vi "Check Settings.vi"(8 "error in (no error)":errorcluster, 10 "Iterator Settings":T1={"Prepare timeout (ms)"=200, "Iterate timeout (ms)"=50, "Conclude timeout (ms)"=200, "Iterate period (ms)"=200, "Number of iterations"=5, "Stop Condition"=enum."None", "Time before stop (ms)"=5, "Prepare Msg"=refnum, "Iterate Msg"=refnum, "Conclude Msg"=refnum, "Error Handler"=refnum}, 11 "Caller Enqueuer in":refnum<class "Message Enqueuer.lvclass">) -> (0 "error out":errorcluster, 3 "Caller Enqueuer out":refnum<class "Message Enqueuer.lvclass">)   [LabVIEW 2016, in "Iterator Actor.lvlib" / "Iterator Actor.lvclass"]
doc: "Checks the input settings of the iterator. \nReturns an error with a description if something is wrong."
uses:
  Iterator Actor.lvclass
  <vilib>/ActorFramework/Message Enqueuer/Message Enqueuer.lvclass
  Iterator Settings.ctl
  Iterator Actor Abstract Messages/Iterator Reply Msg/Iterator Reply Msg.lvclass
  Iterator Actor Abstract Messages/Iterator Report Error Msg/Iterator Report Error Msg.lvclass
  Stop Condition.ctl
  Iterator Errors.ctl
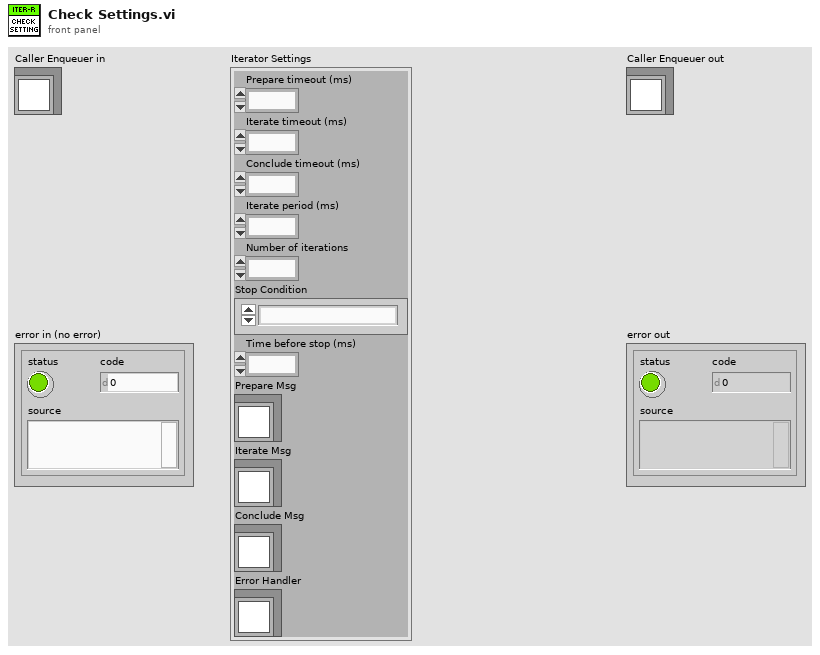
[diagram p1: front panel]
types:
  T1 = typedef "Iterator Actor.lvlib/Iterator Actor.lvclass/Iterator Settings.ctl" = cluster{"Prepare timeout (ms)":i32, "Iterate timeout (ms)":i32, "Conclude timeout (ms)":i32, "Iterate period (ms)":i32, "Number of iterations":i32, "Stop Condition":T2, "Time before stop (ms)":i32, "Prepare Msg":refnum<class "Iterator Reply Msg.lvclass">, "Iterate Msg":refnum<class "Iterator Reply Msg.lvclass">, "Conclude Msg":refnum<class "Iterator Reply Msg.lvclass">, "Error Handler":refnum<class "Iterator Report Error Msg.lvclass">}
  T2 = typedef "Iterator Actor.lvlib/Iterator Actor.lvclass/Stop Condition.ctl" = enum16{"None", "Number of iterations", "Time elapsed", "Iteration result"}
  T3 = typedef "Iterator Actor.lvlib/Iterator Actor.lvclass/Iterator Errors.ctl" = enum16{"Input parameters are not valid", "Preparation call timed out", "Iteration call timed out", "Conclusion call timed out"}
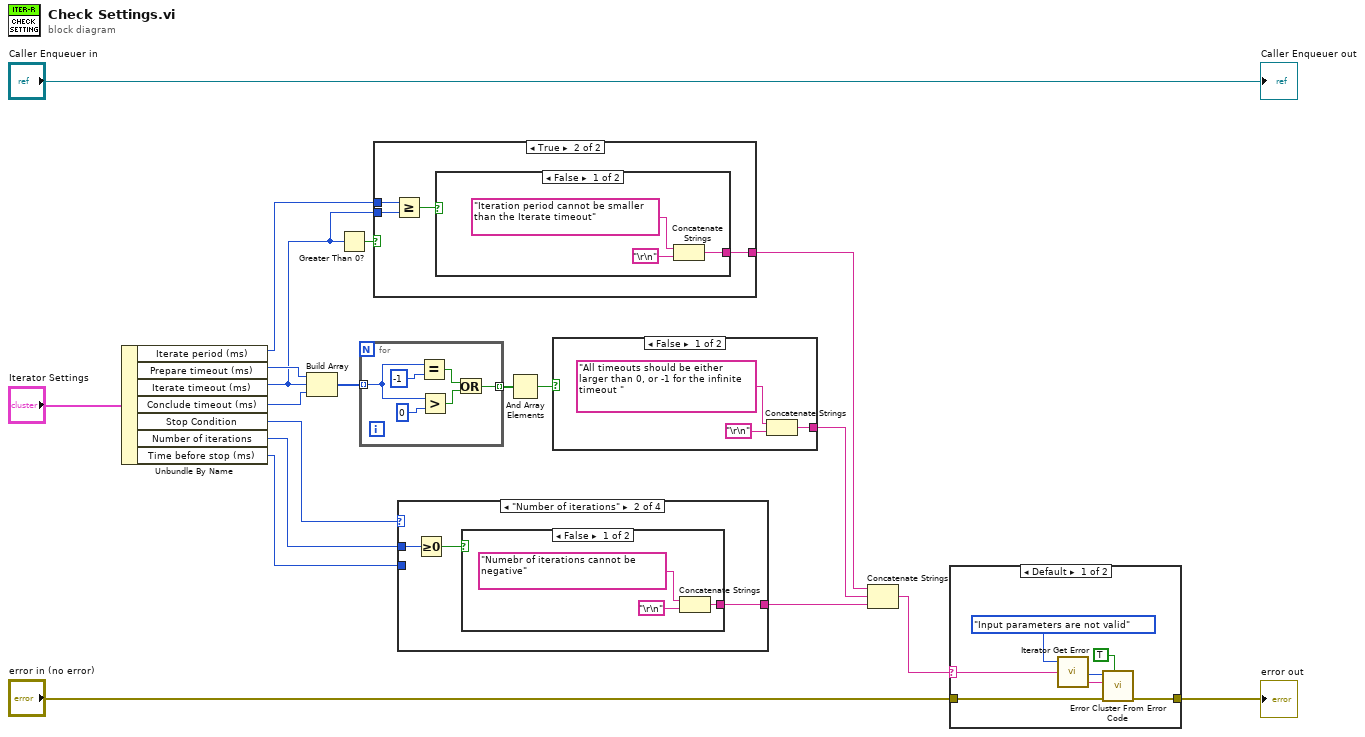
[diagram p0: block diagram]
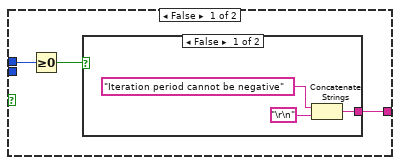
[diagram p2: hidden frame]
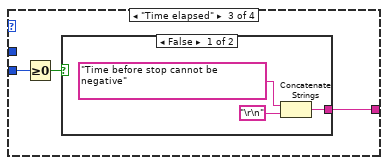
[diagram p9: hidden frame]
diagram:
  n1 = Unbundle By Name("Iterator Settings") -> ("Iterate period (ms)"=w7:i32, "Prepare timeout (ms)"=w14:i32, "Iterate timeout (ms)"=w8:i32, "Conclude timeout (ms)"=w13:i32, "Stop Condition"=w17:T2, "Number of iterations"=w6:i32, "Time before stop (ms)"=w5:i32)
  n2 = Build Array(w14, w8, w13) -> (w12:i32[])
  n3 = Greater Than 0?(x=w8) -> (x > 0?=w9:bool)
  n4 = for {
    tunnel: w12 -> [w23] mode=indexing
    tunnel: [w20] -> w11 mode=indexing
    n5 = Equal?(x=w23, y=-1) -> (x = y?=w21:bool)
    n6 = Greater?(x=w23, y=0) -> (0:w22:bool)
    n7 = Or(x=w21, y=w22) -> (x .or. y?=w20:bool)
  }
  n8 = case shown="True" w9 {
    tunnel: w8 -> [_ w35]
    tunnel: w7 -> [w28 w34]
    tunnel: [w26 w32] -> w2
    frame False {
      n9 = Greater Or Equal To 0?(x=w28) -> (x >= 0?=w27:bool)
      n10 = case shown="False" w27 {
        tunnel: [w30 _] -> w26
        frame False {
          n11 = Concatenate Strings("Iteration period cannot be negative", "\r\n") -> (w30:string)
        }
        frame True {
        }
      }
    }
    frame True {
      n12 = Greater Or Equal?(x=w34, y=w35) -> (x >= y?=w33:bool)
      n13 = case shown="False" w33 {
        tunnel: [w36 _] -> w32
        frame False {
          n14 = Concatenate Strings("Iteration period cannot be smaller than the Iterate timeout", "\r\n") -> (w36:string)
        }
        frame True {
        }
      }
    }
  }
  n15 = case shown="\"Number of iterations\"" w17 {
    tunnel: w6 -> [_ w41 _ _]
    tunnel: w5 -> [_ _ w47 _]
    tunnel: [_ w39 w45 _] -> w4
    frame "None", Default {
    }
    frame "Number of iterations" {
      n16 = Greater Or Equal To 0?(x=w41) -> (x >= 0?=w40:bool)
      n17 = case shown="False" w40 {
        tunnel: [w43 _] -> w39
        frame False {
          n18 = Concatenate Strings("Numebr of iterations cannot be negative", "\r\n") -> (w43:string)
        }
        frame True {
        }
      }
    }
    frame "Time elapsed" {
      n19 = Greater Or Equal To 0?(x=w47) -> (x >= 0?=w46:bool)
      n20 = case shown="False" w46 {
        tunnel: [w48 _] -> w45
        frame False {
          n21 = Concatenate Strings("Time before stop cannot be negative", "\r\n") -> (w48:string)
        }
        frame True {
        }
      }
    }
    frame "Iteration result" {
    }
  }
  n22 = And Array Elements(Boolean array=w11) -> (logical AND=w10:bool)
  n23 = case shown="False" w10 {
    tunnel: [w51 _] -> w3
    frame False {
      n24 = Concatenate Strings("All timeouts should be either larger than 0, or -1 for the infinite timeout ", "\r\n") -> (w51:string)
    }
    frame True {
    }
  }
  n25 = Concatenate Strings(w2, w3, w4) -> (w1:string)
  n26 = case shown="Default" w1 {
    selector: w1 -> [w54 _]
    tunnel: "error in (no error)" -> [w57 w61]
    tunnel: [w56 w61] -> w16
    frame Default {
      n27 = call "Iterator Get Error.vi"("Error Additional Information"=w54, "Error"=Iterator_Errors."Input parameters are not valid") -> ("source"=w59:string, "code"=w58:i32)  [unwired: 1 in, 1 out]
      n28 = call <vilib>:"Error Cluster From Error Code.vi"("show call chain? (False)"=TRUE ("is warning? (False)"), "error in (no error)"=w57, "error message (\"\")"=w59, "error code (0)"=w58) -> ("error out"=w56:errorcluster)  [unwired: 5 in]
    }
    frame "" {
    }
  }
  "error out" <- w16
  "Caller Enqueuer out" <- "Caller Enqueuer in"
